vi "String to number.vi"(1 "positive number string":string) -> (0 "positive value (-1 if invalid)":dbl)   [LabVIEW 2018]
panel:
  # "value RETURNS -1 IF positive number string* CONTAINS ANY CHARACTER \nOTHER THAN [0-9] OR ONE DECIMAL SEPARATOR (COMMA OR POINT)."
  # "(*) after removing white space (spaces, tabs, carriage returns, and linefeeds) from both ends of string."
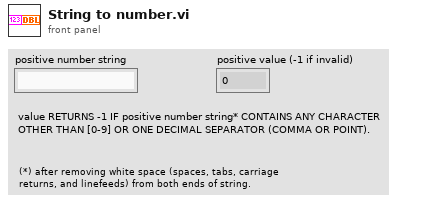
[diagram p1: front panel]
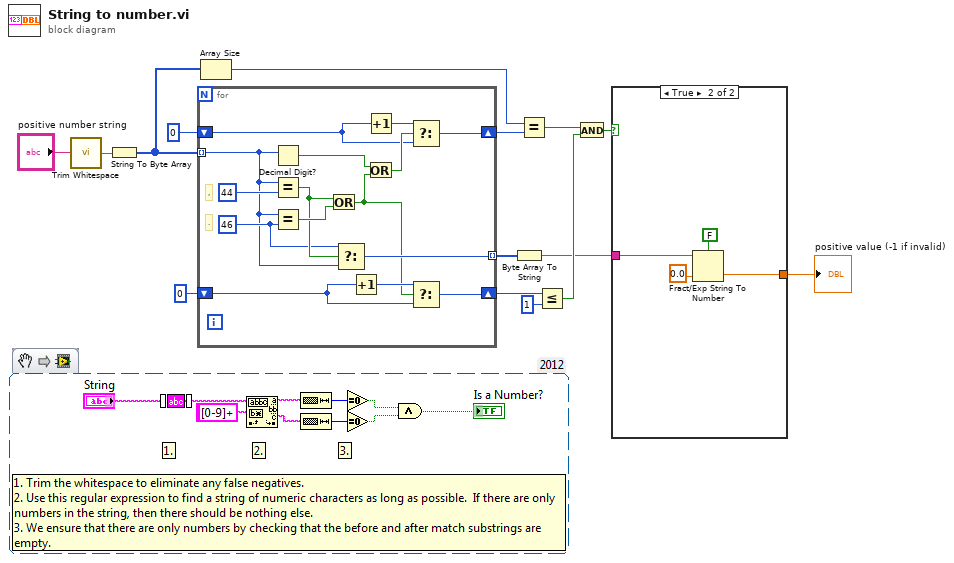
[diagram p0: block diagram]
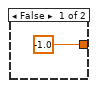
[diagram p2: hidden frame]
diagram:
  n1 = call <vilib>:"Trim Whitespace.vi"("string"="positive number string") -> ("trimmed string"=w13:string)  [unwired: 1 in]
  n2 = String To Byte Array(string=w13) -> (unsigned byte array=w10:u8[])
  n3 = for {
    tunnel: w10 -> [w21] mode=indexing
    shift-right: [w26] -> w6
    shift-left: 0 -> [w24]
    tunnel: [w20] -> w9 mode=indexing
    shift-right: [w18] -> w7
    shift-left: 0 -> [w17]
    w22 = u8 46 ("y")
    # "."
    # ","
    n4 = Decimal Digit?(1:w21) -> (0:w28:bool)
    n5 = Equal?(x=w21, y=u8 44) -> (x = y?=w23:bool)
    n6 = Equal?(x=w21, y=w22) -> (x = y?=w30:bool)
    n7 = Or(x=w23, y=w30) -> (x .or. y?=w16:bool)
    n8 = Select(t=w22, s=w23, f=w21) -> (s? t:f=w20:u8)
    n9 = Increment(x=w17) -> (x+1=w19:i32)
    n10 = Increment(x=w24) -> (x+1=w25:i32)
    n11 = Or(x=w28, y=w16) -> (x .or. y?=w27:bool)
    n12 = Select(t=w25, s=w27, f=w24) -> (s? t:f=w26:i32)
    n13 = Select(t=w19, s=w16, f=w17) -> (s? t:f=w18:i32)
  }
  n14 = Array Size(array=w10) -> (size(s)=w5:i32)
  n15 = Byte Array To String(unsigned byte array=w9) -> (string=w1:string)
  n16 = Equal?(x=w5, y=w6) -> (x = y?=w4:bool)
  n17 = Less Or Equal?(x=w7, y=1) -> (x <= y?=w3:bool)
  n18 = And(x=w4, y=w3) -> (x .and. y?=w2:bool)
  n19 = case shown="True" w2 {
    tunnel: [-1.0 w34] -> w12
    tunnel: w1 -> [_ w32]
    frame False {
    }
    frame True {
      n20 = Fract/Exp String To Number(use system decimal point (T)=FALSE, string=w32, default (0 dbl)=0.0) -> (number=w34:dbl)  [unwired: 1 in, 1 out]
    }
  }
  "positive value (-1 if invalid)" <- w12
